vi "Close.vi"(8 "error in (no error)":errorcluster, 11 "Ismatech 3 Channel Settings In":T1={"VISA resource name"="", "Pump Number"=1, "Channel Number"=0, "Simulated?"=TRUE, "Reverse?"=FALSE} {"Channel Number" min=0 max=3; "Pump Number" min=1 max=9}) -> (0 "error out":errorcluster, 1 "Connection Error":bool, 3 "Ismatech 3 Channel Settings Out":T1={"VISA resource name"="", "Pump Number"=1, "Channel Number"=0, "Simulated?"=TRUE, "Reverse?"=FALSE} {"Channel Number" min=0 max=3; "Pump Number" min=1 max=9})   [LabVIEW 2018, in "Ismatec 4308.lvlib"]
uses:
  Ismatec 4308.lvlib
  Ismatec 4083.ctl
  support/Support Library.lvlib
panel:
  out "read buffer":string
  out "Failed to stop":bool
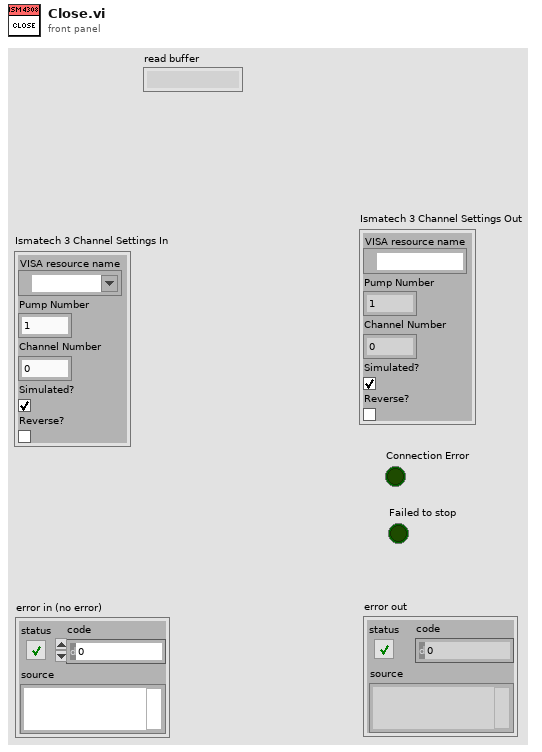
[diagram p1: front panel]
types:
  T1 = typedef "Ismatec 4308.lvlib/Ismatec 4083.ctl" = cluster{"VISA resource name":refnum<visa-resource-name>, "Pump Number":i16, "Channel Number":i16, "Simulated?":bool, "Reverse?":bool}
  T2 = typedef "Ismatec 4308.lvlib/Ismatec 4083 Global.ctl" = T3[]
  T3 = typedef "Ismatec 4308.lvlib/Ismatec 4083 Global Element.ctl" = cluster{"Busy":bool, "ChannelCnt":dbl, "Initialized":bool, "Current Channel":dbl, "Initialized Channels":dbl[]}
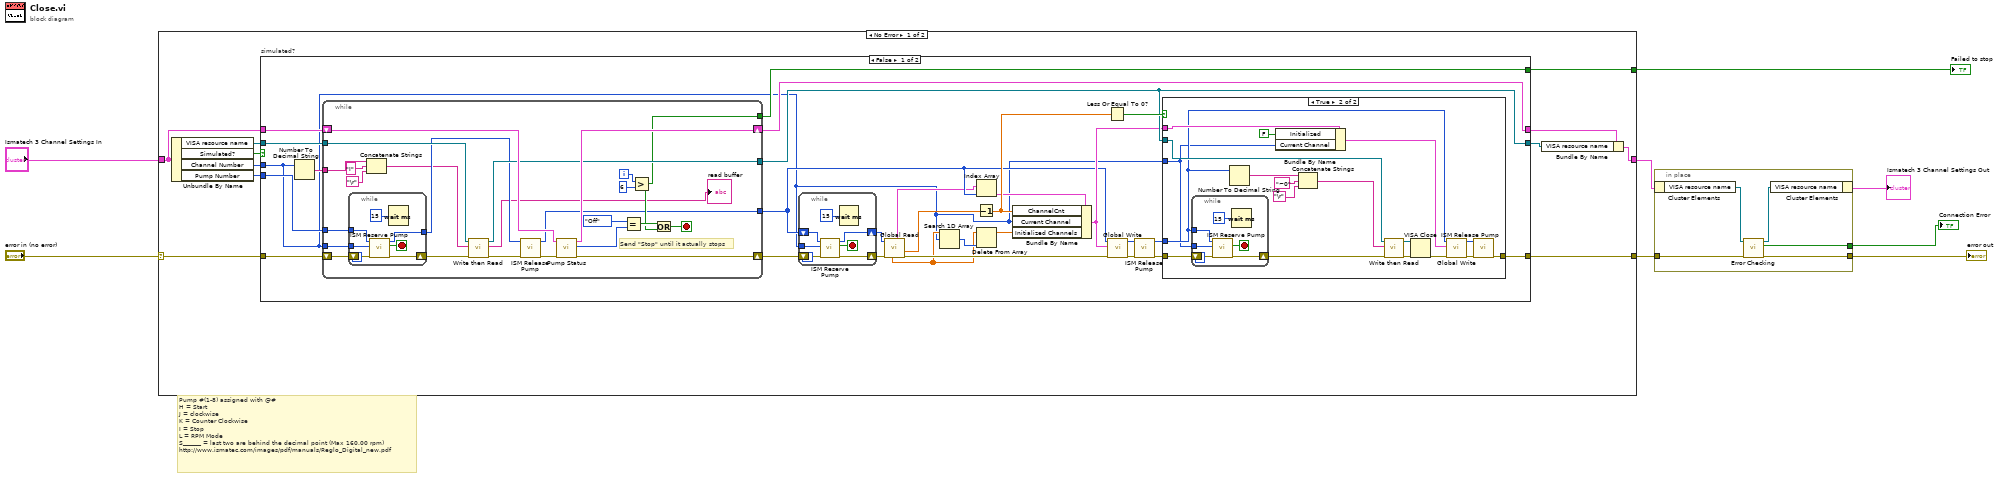
[diagram p0: block diagram]
diagram:
  # "Pump #(1-8) assigned with @#\nH = Start\nJ = clockwise\nK = Counter Clockwise\nI = Stop\nL = RPM Mode\nS______ = last two are behind the decimal point (Max 160.00 rpm)\nhttp://www.ismatec.com/images/pdf/manuals/Reglo_Digital_new.pdf"
  n1 = case shown="No Error" "error in (no error)" {
    selector: "error in (no error)" -> [w14 w116]
    tunnel: [w18 w116] -> w7
    tunnel: [w15 w115] -> w4
    tunnel: "Ismatech 3 Channel Settings In" -> [w11 w115]
    tunnel: [w9 _] -> w1
    frame No Error {
      n2 = Unbundle By Name(w11) -> ("VISA resource name"=w13:refnum<visa-resource-name>, "Simulated?"=w19:bool, "Channel Number"=w16:i16, "Pump Number"=w10:i16)
      n3 = case "simulated?" shown="False" w19 {
        tunnel: [w36 w112] -> w18
        tunnel: [w37 w113] -> w17
        tunnel: w16 -> [w20 _]
        tunnel: w14 -> [w47 w112]
        tunnel: w13 -> [w46 w113]
        tunnel: w11 -> [w45 w114]
        tunnel: [w44 w114] -> w12
        tunnel: w10 -> [w28 _]
        tunnel: [w42 _] -> w9
        frame False {
          n4 = Number To Decimal String(number=w20) -> (decimal integer string=w43:string)  [unwired: 1 in]
          n5 = while {
            tunnel: w46 -> [w102]
            shift-right: [w103] -> w35
            shift-left: w47 -> [w95]
            shift-right: [w100] -> w44
            shift-left: w45 -> [w101]
            tunnel: [w98] -> w37
            tunnel: w43 -> [w96]
            tunnel: w28 -> [w94]
            tunnel: [w89] -> w42
            tunnel: [w83] -> w25
            tunnel: w20 -> [w82]
            i -> [w81]
            stop <- w90 stop-if-true
            # "Send \"Stop\" until it actually stops"
            n6 = while {
              tunnel: w94 -> [w110]
              tunnel: [w108] -> w92
              tunnel: w82 -> [w107]
              shift-right: [w109] -> w93
              shift-left: w95 -> [w111]
              stop <- w105 stop-if-true
              n7 = call "ISM Reserve Pump.vi"("error in (no error)"=w111, "ISM Channel # In"=w107, "ISM Pump # In"=w110) -> ("error out"=w109:errorcluster, "Loop Completed"=w105:bool, "ISM Pump # Out"=w108:i32)  [unwired: 6 in]
              n8 = Wait (ms)(milliseconds to wait=u32 15) -> ()  [unwired: 1 out]
            }
            n9 = Concatenate Strings(w96, "I" ("string"), "\r") -> (w86:string)
            n10 = call "Write then Read.vi"("error in"=w93, "write buffer"=w86, "VISA resource name in"=w102) -> ("error out"=w85:errorcluster, "read buffer"=→"read buffer":string, "VISA resource name out"=w98:refnum<visa-resource-name>)  [unwired: 5 in, 1 out]
            n11 = call "ISM Release Pump.vi"("error in (no error)"=w85, "Pump Number In"=w92) -> ("error out"=w104:errorcluster, "Pump Number Out"=w83:i32)  [unwired: 8 in]
            n12 = call "Pump Status.vi"("error in (no error)"=w104, "Ismatech 3 Channel Settings In"=w101) -> ("error out"=w103:errorcluster, "Pump On?"=w99:enum16{"Off", "On", "Not Initialized"}, "Ismatech 3 Channel Settings Out"=w100:T1)  [unwired: 5 in, 2 out]
            n13 = Equal?(x=enum16{"Off", "On", "Not Initialized"}."Off", y=w99) -> (x = y?=w91:bool)
            n14 = Greater?(x=w81, y=6 ("x")) -> (0:w89:bool)
            n15 = Or(x=w91, y=w89) -> (x .or. y?=w90:bool)
          }
          n16 = while {
            tunnel: w20 -> [w50]
            shift-right: [w52] -> w33
            shift-left: w35 -> [w54]
            shift-right: [w53] -> w34
            shift-left: w25 -> [w51]
            stop <- w49 stop-if-true
            n17 = call "ISM Reserve Pump.vi"("error in (no error)"=w54, "ISM Channel # In"=w50, "ISM Pump # In"=w51) -> ("error out"=w52:errorcluster, "Loop Completed"=w49:bool, "ISM Pump # Out"=w53:i32)  [unwired: 6 in]
            n18 = Wait (ms)(milliseconds to wait=u32 15) -> ()  [unwired: 1 out]
          }
          n19 = call "Global Read.vi"("error in (no error)"=w33, "Pump Number"=w34) -> ("error out"=w40:errorcluster, "ChannelCnt"=w41:dbl, "Ismatec 4083 Global"=w24:T2, "Initialized Channels"=w21:dbl[])  [unwired: 3 in, 3 out]
          n20 = Search 1D Array(1D array=w21, element=w20) -> (index of element=w22:i32)  [unwired: 1 in]
          n21 = Index Array(array=w24, index=w25) -> (element=w27:T3)
          n22 = Decrement(x=w41) -> (x-1=w38:dbl)
          n23 = Delete From Array(array=w21, index=w22) -> (array with subset deleted=w23:dbl[])  [unwired: 1 in, 1 out]
          n24 = Bundle By Name(cluster=w27, "ChannelCnt"=w38, "Current Channel"=w20, "Initialized Channels"=w23) -> (w26:T3)
          n25 = Less Or Equal To 0?(x=w38) -> (x <= 0?=w39:bool)
          n26 = call "Global Write.vi"("error in (no error)"=w40, "Incoming Cluster"=w26, "Pump Number In"=w25) -> ("error out"=w31:errorcluster, "Pump Number Out"=w32:i32)  [unwired: 7 in]
          n27 = call "ISM Release Pump.vi"("error in (no error)"=w31, "Pump Number In"=w32) -> ("error out"=w30:errorcluster, "Pump Number Out"=w29:i32)  [unwired: 8 in]
          n28 = case shown="True" w39 {
            tunnel: w29 -> [_ w58]
            tunnel: w37 -> [_ w63]
            tunnel: w30 -> [w55 w60]
            tunnel: [w55 w65] -> w36
            tunnel: w26 -> [_ w68]
            tunnel: w20 -> [_ w56]
            frame False {
            }
            frame True {
              n29 = while {
                tunnel: w58 -> [w77]
                tunnel: w56 -> [w76]
                shift-right: [w78] -> w59
                shift-left: w60 -> [w79]
                stop <- w75 stop-if-true
                n30 = call "ISM Reserve Pump.vi"("error in (no error)"=w79, "ISM Channel # In"=w76, "ISM Pump # In"=w77) -> ("error out"=w78:errorcluster, "Loop Completed"=w75:bool)  [unwired: 6 in, 1 out]
                n31 = Wait (ms)(milliseconds to wait=u32 15) -> ()  [unwired: 1 out]
              }
              n32 = Number To Decimal String(number=w58) -> (decimal integer string=w71:string)  [unwired: 1 in]
              n33 = Bundle By Name(cluster=w68, "Initialized"=FALSE, "Current Channel"=w56) -> (w66:T3)
              n34 = Concatenate Strings(w71, "~0" ("string"), "\r") -> (w64:string)
              n35 = call "Write then Read.vi"("error in"=w59, "write buffer"=w64, "VISA resource name in"=w63) -> ("error out"=w61:errorcluster, "VISA resource name out"=w62:refnum<visa-resource-name>)  [unwired: 5 in, 2 out]
              n36 = VISA Close(VISA resource name=w62, error in (no error)=w61) -> (error out=w57:errorcluster)
              n37 = call "Global Write.vi"("error in (no error)"=w57, "Incoming Cluster"=w66, "Pump Number In"=w58) -> ("error out"=w70:errorcluster, "Pump Number Out"=w69:i32)  [unwired: 7 in]
              n38 = call "ISM Release Pump.vi"("error in (no error)"=w70, "Pump Number In"=w69) -> ("error out"=w65:errorcluster)  [unwired: 8 in, 1 out]
            }
          }
        }
        frame True {
        }
      }
      n39 = Bundle By Name(cluster=w12, "VISA resource name"=w17) -> (w15:T1)
    }
    frame Error {
    }
  }
  "Failed to stop" <- w1
  n40 = in-place {
    in-place-border: w7 -> [w121]
    in-place-border: [w120] -> w6
    in-place-border: [w119] -> w5
    n41 = in-place-cluster #1(w4) -> ("VISA resource name"=w118:refnum<visa-resource-name>)
    n42 = call "Error Checking.vi"("error in (no error)"=w121, "VISA resource name"=w118) -> ("error out"=w120:errorcluster, "Connection Error"=w119:bool, "VISA resource name"=w117:refnum<visa-resource-name>)  [unwired: 7 in]
    n43 = in-place-cluster #1("VISA resource name"=w117) -> (→"Ismatech 3 Channel Settings Out":T1)
  }
  "error out" <- w6
  "Connection Error" <- w5
